vi "RW PI Info.vi"(0 "Refnum In":T2, 2 "Read (F)":bool, 7 "PIinfo In":T1(array[cluster]), 11 "Error In":errorcluster) -> (4 "Refnum Out":T2, 8 "PIinfo Out":T1(array[cluster]), 15 "Error Out":errorcluster)   [LabVIEW 2013]
uses:
  <vilib>/Utility/config.llb/Config Data RefNum.ctl
  <vilib>/Utility/config.llb/Write Key (Double).vi
  <vilib>/Utility/config.llb/Read Key (Double).vi
  <vilib>/Utility/config.llb/NI_LVConfig.lvlib
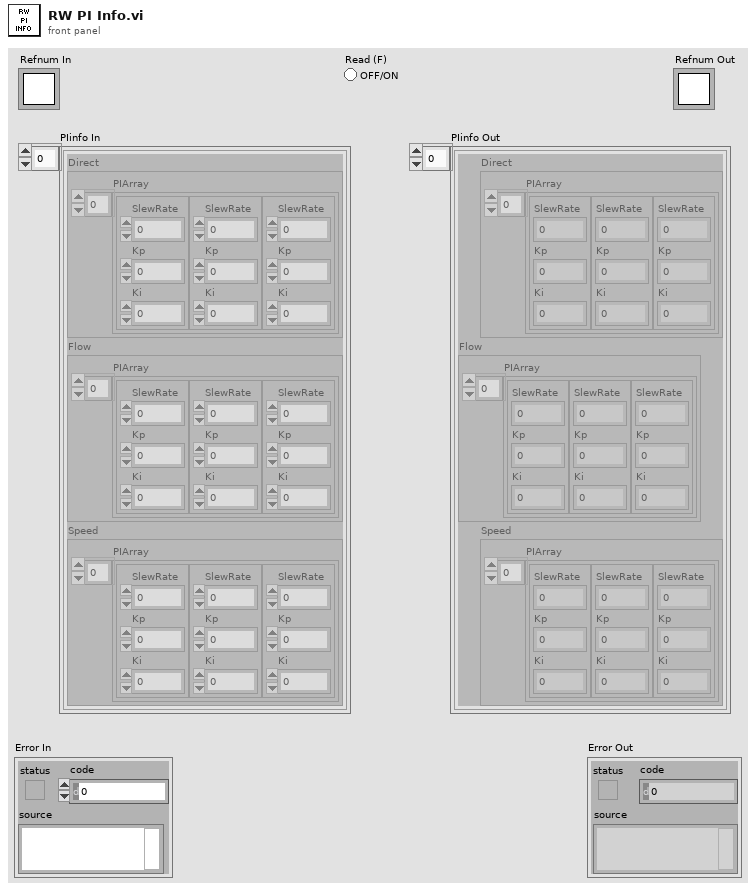
[diagram p1: front panel]
types:
  T1 = cluster{"Direct":cluster{"PIArray":cluster{"SlewRate":dbl, "Kp":dbl, "Ki":dbl}[]}, "Flow":cluster{"PIArray":cluster{"SlewRate":dbl, "Kp":dbl, "Ki":dbl}[]}, "Speed":cluster{"PIArray":cluster{"SlewRate":dbl, "Kp":dbl, "Ki":dbl}[]}}[]
  T2 = typedef "NI_LVConfig.lvlib/Config Data RefNum.ctl" = refnum<k1>
  T3 = cluster{"Direct":cluster{"PIArray":cluster{"SlewRate":dbl, "Kp":dbl, "Ki":dbl}[]}, "Flow":cluster{"PIArray":cluster{"SlewRate":dbl, "Kp":dbl, "Ki":dbl}[]}, "Speed":cluster{"PIArray":cluster{"SlewRate":dbl, "Kp":dbl, "Ki":dbl}[]}}
  T4 = cluster{"PIArray":cluster{"SlewRate":dbl, "Kp":dbl, "Ki":dbl}[]}
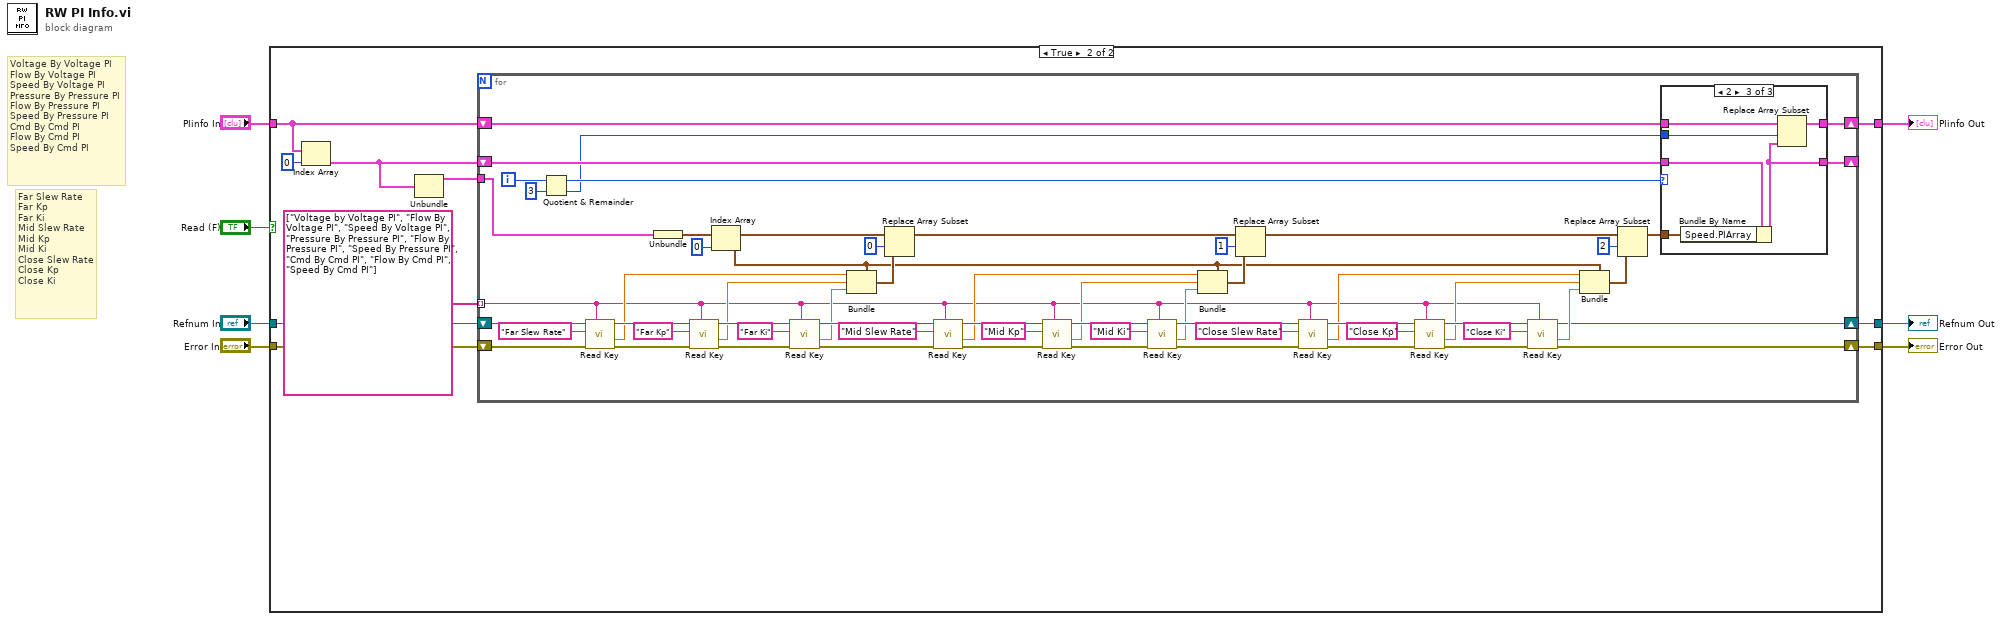
[diagram p0: block diagram]
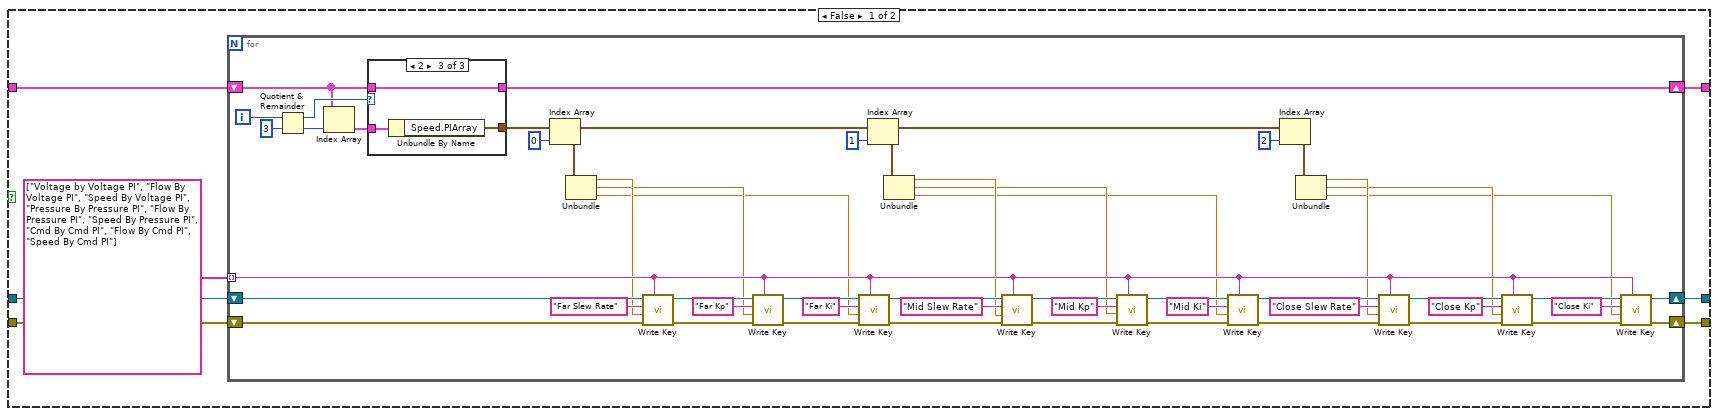
[diagram p2: hidden frame]
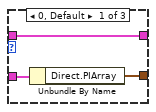
[diagram p3: hidden frame]
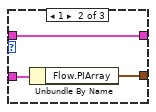
[diagram p4: hidden frame]
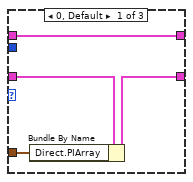
[diagram p5: hidden frame]
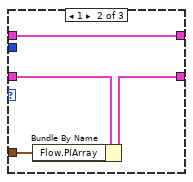
[diagram p6: hidden frame]
diagram:
  # "Far Slew Rate\nFar Kp\nFar Ki\nMid Slew Rate\nMid Kp\nMid Ki\nClose Slew Rate\nClose Kp\nClose Ki"
  # "Voltage By Voltage PI\nFlow By Voltage PI\nSpeed By Voltage PI\nPressure By Pressure PI\nFlow By Pressure PI\nSpeed By Pressure PI\nCmd By Cmd PI\nFlow By Cmd PI\nSpeed By Cmd PI"
  n1 = case shown="True" "Read (F)" {
    tunnel: "Error In" -> [w12 w85]
    tunnel: [w8 w82] -> w6
    tunnel: "Refnum In" -> [w11 w86]
    tunnel: [w9 w83] -> w3
    tunnel: "PIinfo In" -> [w13 w80]
    tunnel: [w10 w79] -> w2
    frame False {
      n2 = for {
        shift-right: [w43] -> w9
        shift-left: w11 -> [w52]
        shift-right: [w53] -> w8
        shift-left: w12 -> [w62]
        tunnel: string[] ["Voltage by Voltage PI", "Flow By Voltage PI", "Speed By Voltage PI", "Pressure By Pressure PI", "Flow By Pressure PI", "Speed By Pressure PI", "Cmd By Cmd PI", "Flow By Cmd PI", "Speed By Cmd PI"] -> [w33] mode=indexing
        shift-right: [w63] -> w10
        shift-left: w13 -> [w31]
        i -> [w66]
        n3 = Quotient & Remainder(x=w66, y=3) -> (x-y*floor(x/y)=w64:i32, floor(x/y)=w32:i32)
        n4 = Index Array(array=w31, index=w32) -> (element=w30:T3)
        n5 = case shown="2" w64 {
          tunnel: w30 -> [w69 w72 w75]
          tunnel: w31 -> [w70 w73 w76]
          tunnel: [w70 w73 w76] -> w63
          tunnel: [w68 w71 w74] -> w27
          frame 0, Default {
            n6 = Unbundle By Name(w69) -> ("Direct.PIArray"=w68:cluster{"SlewRate":dbl, "Kp":dbl, "Ki":dbl}[])
          }
          frame 1 {
            n7 = Unbundle By Name(w72) -> ("Flow.PIArray"=w71:cluster{"SlewRate":dbl, "Kp":dbl, "Ki":dbl}[])
          }
          frame 2 {
            n8 = Unbundle By Name(w75) -> ("Speed.PIArray"=w74:cluster{"SlewRate":dbl, "Kp":dbl, "Ki":dbl}[])
          }
        }
        n9 = Index Array(array=w27, index=0) -> (element=w26:cluster{"SlewRate":dbl, "Kp":dbl, "Ki":dbl})
        n10 = Unbundle(w26) -> ("SlewRate"=w23:dbl, "Kp"=w22:dbl, "Ki"=w21:dbl)
        n11 = call-poly <vilib>:"Write Key.vi"("section"=w33, "error in (no error)"=w62, "value"=w23, "key"="Far Slew Rate", "refnum"=w52) -> ("error out"=w61:errorcluster, "refnum out"=w51:T2)  [unwired: 4 in, 1 out]
        n12 = call-poly <vilib>:"Write Key.vi"("section"=w33, "error in (no error)"=w61, "value"=w22, "key"="Far Kp", "refnum"=w51) -> ("error out"=w60:errorcluster, "refnum out"=w50:T2)  [unwired: 4 in, 1 out]
        n13 = call-poly <vilib>:"Write Key.vi"("section"=w33, "error in (no error)"=w60, "value"=w21, "key"="Far Ki", "refnum"=w50) -> ("error out"=w59:errorcluster, "refnum out"=w49:T2)  [unwired: 4 in, 1 out]
        n14 = Index Array(array=w27, index=1) -> (element=w25:cluster{"SlewRate":dbl, "Kp":dbl, "Ki":dbl})
        n15 = Unbundle(w25) -> ("SlewRate"=w17:dbl, "Kp"=w16:dbl, "Ki"=w15:dbl)
        n16 = call-poly <vilib>:"Write Key.vi"("section"=w33, "error in (no error)"=w59, "value"=w17, "key"="Mid Slew Rate", "refnum"=w49) -> ("error out"=w58:errorcluster, "refnum out"=w48:T2)  [unwired: 4 in, 1 out]
        n17 = call-poly <vilib>:"Write Key.vi"("section"=w33, "error in (no error)"=w58, "value"=w16, "key"="Mid Kp", "refnum"=w48) -> ("error out"=w57:errorcluster, "refnum out"=w47:T2)  [unwired: 4 in, 1 out]
        n18 = call-poly <vilib>:"Write Key.vi"("section"=w33, "error in (no error)"=w57, "value"=w15, "key"="Mid Ki", "refnum"=w47) -> ("error out"=w56:errorcluster, "refnum out"=w46:T2)  [unwired: 4 in, 1 out]
        n19 = Index Array(array=w27, index=2) -> (element=w24:cluster{"SlewRate":dbl, "Kp":dbl, "Ki":dbl})
        n20 = Unbundle(w24) -> ("SlewRate"=w20:dbl, "Kp"=w19:dbl, "Ki"=w18:dbl)
        n21 = call-poly <vilib>:"Write Key.vi"("section"=w33, "error in (no error)"=w56, "value"=w20, "key"="Close Slew Rate", "refnum"=w46) -> ("error out"=w55:errorcluster, "refnum out"=w45:T2)  [unwired: 4 in, 1 out]
        n22 = call-poly <vilib>:"Write Key.vi"("section"=w33, "error in (no error)"=w55, "value"=w19, "key"="Close Kp", "refnum"=w45) -> ("error out"=w54:errorcluster, "refnum out"=w44:T2)  [unwired: 4 in, 1 out]
        n23 = call-poly <vilib>:"Write Key.vi"("section"=w33, "error in (no error)"=w54, "value"=w18, "key"="Close Ki", "refnum"=w44) -> ("error out"=w53:errorcluster, "refnum out"=w43:T2)  [unwired: 4 in, 1 out]
      }
    }
    frame True {
      n24 = Index Array(array=w80, index=0) -> (element=w78:T3)
      n25 = Unbundle(w78) -> ("Direct"=w77:T4)  [unwired: 2 out]
      n26 = for {
        shift-right: [w99] -> w83
        shift-left: w86 -> [w146]
        shift-right: [w98] -> w82
        shift-left: w85 -> [w145]
        tunnel: string[] ["Voltage by Voltage PI", "Flow By Voltage PI", "Speed By Voltage PI", "Pressure By Pressure PI", "Flow By Pressure PI", "Speed By Pressure PI", "Cmd By Cmd PI", "Flow By Cmd PI", "Speed By Cmd PI"] -> [w97] mode=indexing
        shift-right: [w91] -> _
        shift-left: w78 -> [w92]
        shift-right: [w89] -> w79
        shift-left: w80 -> [w90]
        tunnel: w77 -> [w87]
        i -> [w96]
        n27 = Quotient & Remainder(x=w96, y=3) -> (x-y*floor(x/y)=w94:i32, floor(x/y)=w88:i32)
        n28 = call-poly <vilib>:"Read Key.vi"("section"=w97, "error in (no error)"=w145, "key"="Far Slew Rate", "refnum"=w146) -> ("error out"=w129:errorcluster, "value"=w108:dbl, "refnum out"=w144:T2)  [unwired: 4 in, 1 out]
        n29 = Unbundle(w87) -> ("PIArray"=w117:cluster{"SlewRate":dbl, "Kp":dbl, "Ki":dbl}[])
        n30 = call-poly <vilib>:"Read Key.vi"("section"=w97, "error in (no error)"=w129, "key"="Far Kp", "refnum"=w144) -> ("error out"=w130:errorcluster, "value"=w107:dbl, "refnum out"=w143:T2)  [unwired: 4 in, 1 out]
        n31 = Index Array(array=w117, index=0) -> (element=w109:cluster{"SlewRate":dbl, "Kp":dbl, "Ki":dbl})
        n32 = call-poly <vilib>:"Read Key.vi"("section"=w97, "error in (no error)"=w130, "key"="Far Ki", "refnum"=w143) -> ("error out"=w131:errorcluster, "value"=w106:dbl, "refnum out"=w142:T2)  [unwired: 4 in, 1 out]
        n33 = Bundle(cluster=w109, "SlewRate"=w108, "Kp"=w107, "Ki"=w106) -> (w116:cluster{"SlewRate":dbl, "Kp":dbl, "Ki":dbl})
        n34 = Replace Array Subset(array=w117, new element=w116, index=0) -> (w113:cluster{"SlewRate":dbl, "Kp":dbl, "Ki":dbl}[])
        n35 = call-poly <vilib>:"Read Key.vi"("section"=w97, "error in (no error)"=w131, "key"="Mid Slew Rate", "refnum"=w142) -> ("error out"=w132:errorcluster, "value"=w105:dbl, "refnum out"=w141:T2)  [unwired: 4 in, 1 out]
        n36 = call-poly <vilib>:"Read Key.vi"("section"=w97, "error in (no error)"=w132, "key"="Mid Kp", "refnum"=w141) -> ("error out"=w133:errorcluster, "value"=w104:dbl, "refnum out"=w140:T2)  [unwired: 4 in, 1 out]
        n37 = call-poly <vilib>:"Read Key.vi"("section"=w97, "error in (no error)"=w133, "key"="Mid Ki", "refnum"=w140) -> ("error out"=w134:errorcluster, "value"=w103:dbl, "refnum out"=w139:T2)  [unwired: 4 in, 1 out]
        n38 = Bundle(cluster=w109, "SlewRate"=w105, "Kp"=w104, "Ki"=w103) -> (w111:cluster{"SlewRate":dbl, "Kp":dbl, "Ki":dbl})
        n39 = Replace Array Subset(array=w113, new element=w111, index=1) -> (w112:cluster{"SlewRate":dbl, "Kp":dbl, "Ki":dbl}[])
        n40 = call-poly <vilib>:"Read Key.vi"("section"=w97, "error in (no error)"=w134, "key"="Close Slew Rate", "refnum"=w139) -> ("error out"=w135:errorcluster, "value"=w102:dbl, "refnum out"=w138:T2)  [unwired: 4 in, 1 out]
        n41 = call-poly <vilib>:"Read Key.vi"("section"=w97, "error in (no error)"=w135, "key"="Close Kp", "refnum"=w138) -> ("error out"=w136:errorcluster, "value"=w101:dbl, "refnum out"=w137:T2)  [unwired: 4 in, 1 out]
        n42 = call-poly <vilib>:"Read Key.vi"("section"=w97, "error in (no error)"=w136, "key"="Close Ki", "refnum"=w137) -> ("error out"=w98:errorcluster, "value"=w100:dbl, "refnum out"=w99:T2)  [unwired: 4 in, 1 out]
        n43 = Bundle(cluster=w109, "SlewRate"=w102, "Kp"=w101, "Ki"=w100) -> (w110:cluster{"SlewRate":dbl, "Kp":dbl, "Ki":dbl})
        n44 = Replace Array Subset(array=w112, new element=w110, index=2) -> (w93:cluster{"SlewRate":dbl, "Kp":dbl, "Ki":dbl}[])
        n45 = case shown="2" w94 {
          tunnel: w92 -> [w150 w154 w160]
          tunnel: w93 -> [w149 w153 w159]
          tunnel: [w148 w152 w155] -> w91
          tunnel: w90 -> [w147 w151 w158]
          tunnel: [w147 w151 w157] -> w89
          tunnel: w88 -> [_ _ w156]
          frame 0, Default {
            n46 = Bundle By Name(cluster=w150, "Direct.PIArray"=w149) -> (w148:T3)
          }
          frame 1 {
            n47 = Bundle By Name(cluster=w154, "Flow.PIArray"=w153) -> (w152:T3)
          }
          frame 2 {
            n48 = Bundle By Name(cluster=w160, "Speed.PIArray"=w159) -> (w155:T3)
            n49 = Replace Array Subset(array=w158, new element=w155, index=w156) -> (w157:T1)
          }
        }
      }
    }
  }
  "Refnum Out" <- w3
  "Error Out" <- w6
  "PIinfo Out" <- w2
